vi "volt_curr_CH1_CH2_to_indicators.vi"(9 "CH1 / CH2":bool, 10 "Volt / Curr":bool, 11 "Knob":dbl(knob) scale=0.0..10.0) -> (0 "Current Target CH2":dbl, 1 "Voltage  Target CH2":dbl, 2 "Curent Target CH1":dbl, 3 "Voltage Target CH1":dbl)   [LabVIEW 2020]
doc: "przypisuje wartość numeryczną w zależności od ustawień dwuch przełączników bool"
panel:
  out "CH1 / CH2":bool
  out "Voltage / Curr":bool
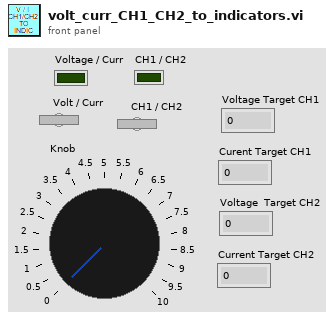
[diagram p1: front panel]
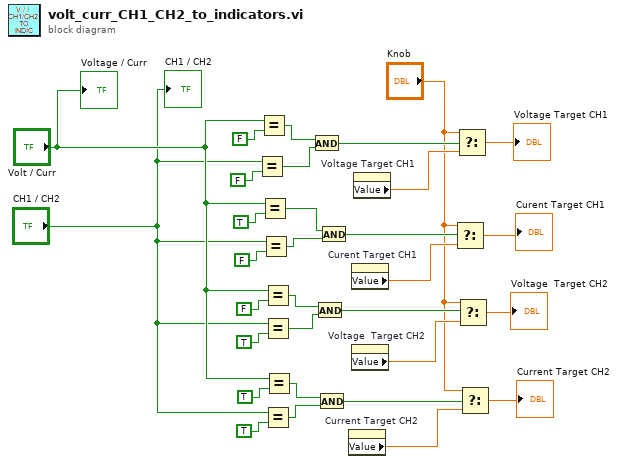
[diagram p0: block diagram]
diagram:
  n1 = Equal?(x="CH1 / CH2", y=FALSE) -> (x = y?=w22:bool)
  n2 = Equal?(x="Volt / Curr", y=FALSE) -> (x = y?=w23:bool)
  n3 = Equal?(x="Volt / Curr", y=TRUE) -> (x = y?=w21:bool)
  n4 = Equal?(x="CH1 / CH2", y=FALSE) -> (x = y?=w20:bool)
  n5 = Equal?(x="Volt / Curr", y=FALSE) -> (x = y?=w19:bool)
  n6 = Equal?(x="CH1 / CH2", y=TRUE) -> (x = y?=w18:bool)
  n7 = Equal?(x="CH1 / CH2", y=TRUE) -> (x = y?=w16:bool)
  n8 = Equal?(x="Volt / Curr", y=TRUE) -> (x = y?=w17:bool)
  n9 = And(x=w23, y=w22) -> (x .and. y?=w15:bool)
  n10 = And(x=w19, y=w18) -> (x .and. y?=w13:bool)
  n11 = And(x=w17, y=w16) -> (x .and. y?=w14:bool)
  n12 = And(x=w21, y=w20) -> (x .and. y?=w12:bool)
  n13 = property on="Current Target CH2" class="DigNum (strict)"() -> ("Value"=w4:dbl)  [unwired: 2 in, 2 out]
  n14 = property on="Curent Target CH1" class="DigNum (strict)"() -> ("Value"=w6:dbl)  [unwired: 2 in, 2 out]
  n15 = property on="Voltage  Target CH2" class="DigNum (strict)"() -> ("Value"=w5:dbl)  [unwired: 2 in, 2 out]
  n16 = property on="Voltage Target CH1" class="DigNum (strict)"() -> ("Value"=w7:dbl)  [unwired: 2 in, 2 out]
  n17 = Select(t="Knob", s=w12, f=w6) -> (s? t:f=→"Curent Target CH1":dbl)
  n18 = Select(t="Knob", s=w15, f=w7) -> (s? t:f=→"Voltage Target CH1":dbl)
  n19 = Select(t="Knob", s=w13, f=w5) -> (s? t:f=→"Voltage  Target CH2":dbl)
  n20 = Select(t="Knob", s=w14, f=w4) -> (s? t:f=→"Current Target CH2":dbl)
  "Voltage / Curr" <- "Volt / Curr"
  "CH1 / CH2" <- "CH1 / CH2"
